vi "main 7th.vi"() -> ()   [LabVIEW 2015]
panel:
  out "3":u32
  out "1":u32
  out "2":u32
  out "5":u32
  out "4":u32
  out "element":u16[][](array[numeric])
  out "From OD fit?":bool
  in  "Current file num":i32
  in  "Fitting Results Save Path":string[](array[string])
  in  "Initial guess values":dbl[](array[numeric])
  out "Latest image data":dbl[][](array[numeric])
  in  "Fitting Type":u16(ring)
  in  "Force Guess?":bool
  in  "milliseconds to wait":u32
  out "best fit parameters":dbl[](array[numeric])
  in  "Reset process index":bool
  out "ROI Height":u32
  out "ROI Width":u32
  out "OD image":u16[][](graph)
  out "Process Index":i32
  out "External Trigger":bool
  out "XY图":cluster{i32[], dbl[]}[](graph)
  in  "OD fit":bool
  in  "OD num":i32
  out "Fit Done":bool
  in  "Exit":bool
  out "XY图 2":cluster{i32[], dbl[]}[](graph)
  in  "Fit":bool
  in  "Open File":bool
  in  "Auto Fit":bool
  in  "Stop":bool
  in  "Aquire":bool
  in  "Fitting Config":bool
  in  "Camera Config":bool
  in  "Initialize":bool
  in  "Live Image Display":refnum<k7>(container)
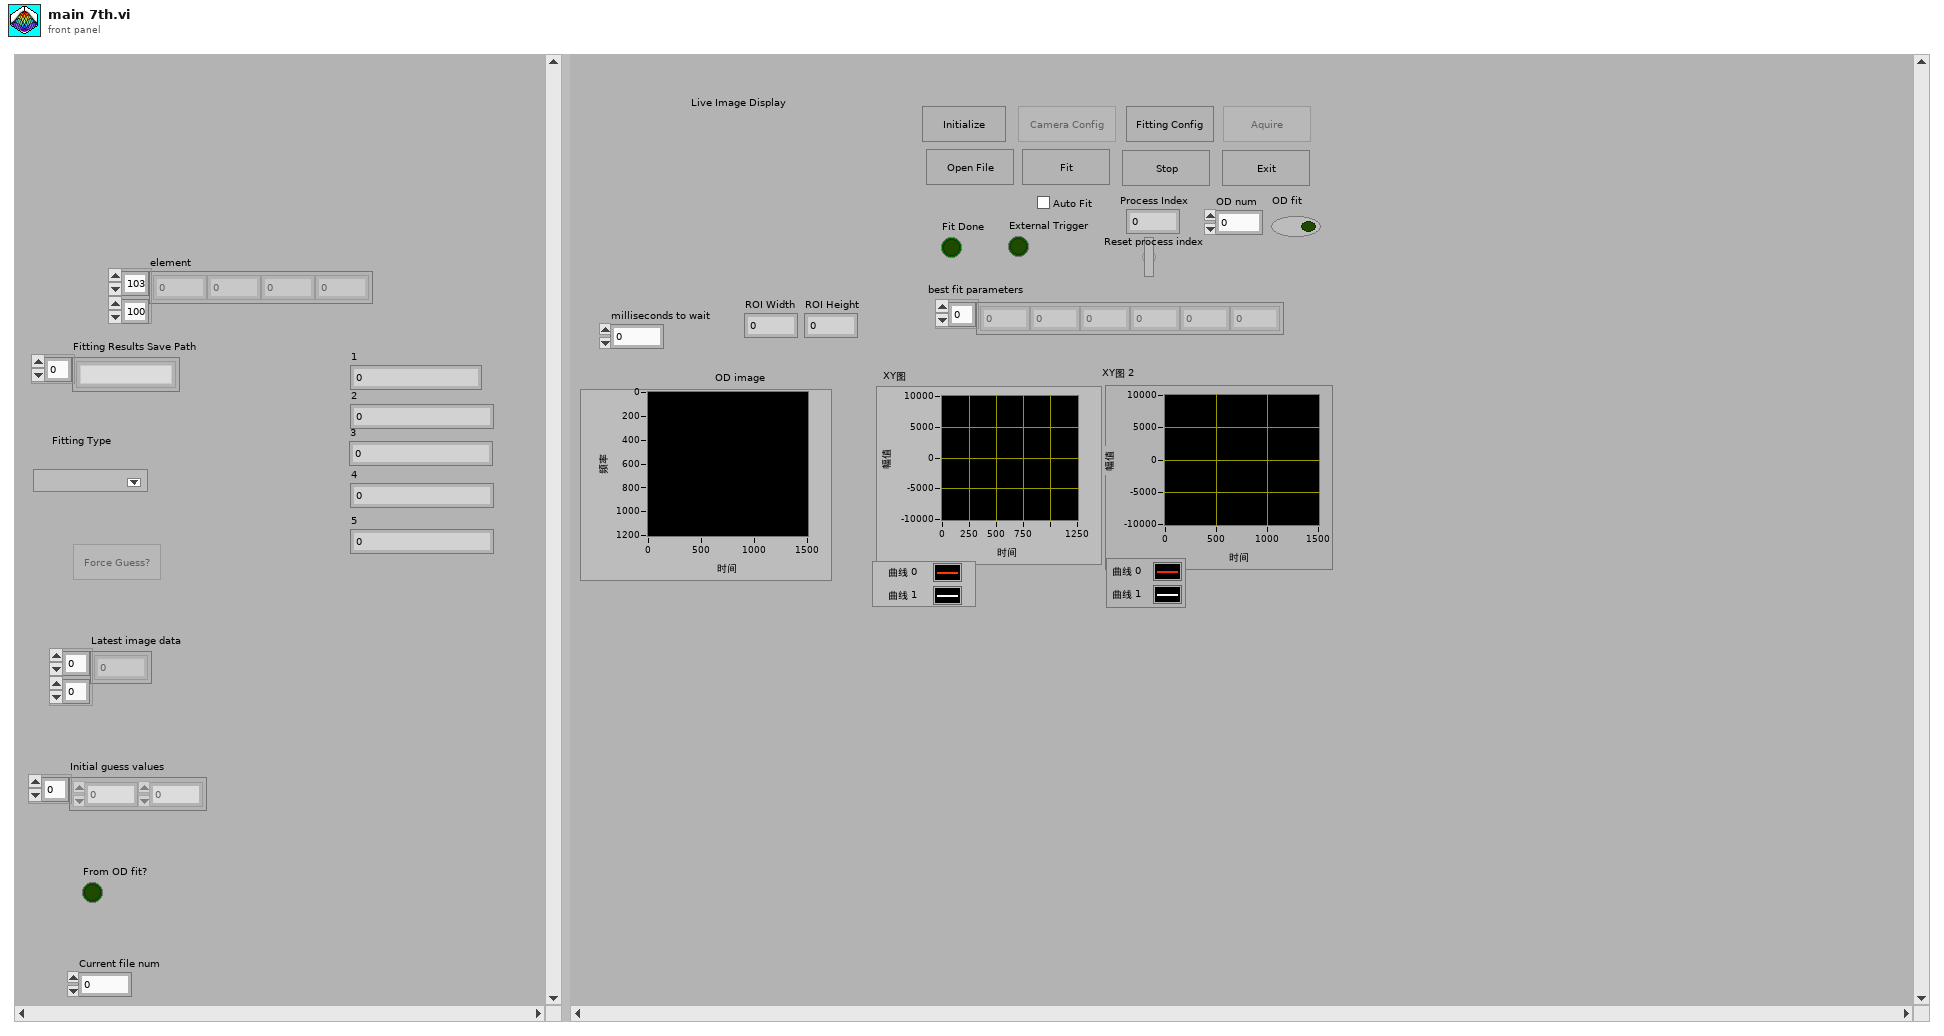
[diagram p1: front panel]
types:
  T1 = enum8{"Enabled", "Disabled", "Disabled and Grayed Out"}
  T2 = typedef "Image Type" = u32
  T3 = typedef "IMAQ Image.ctl" = refnum<image>
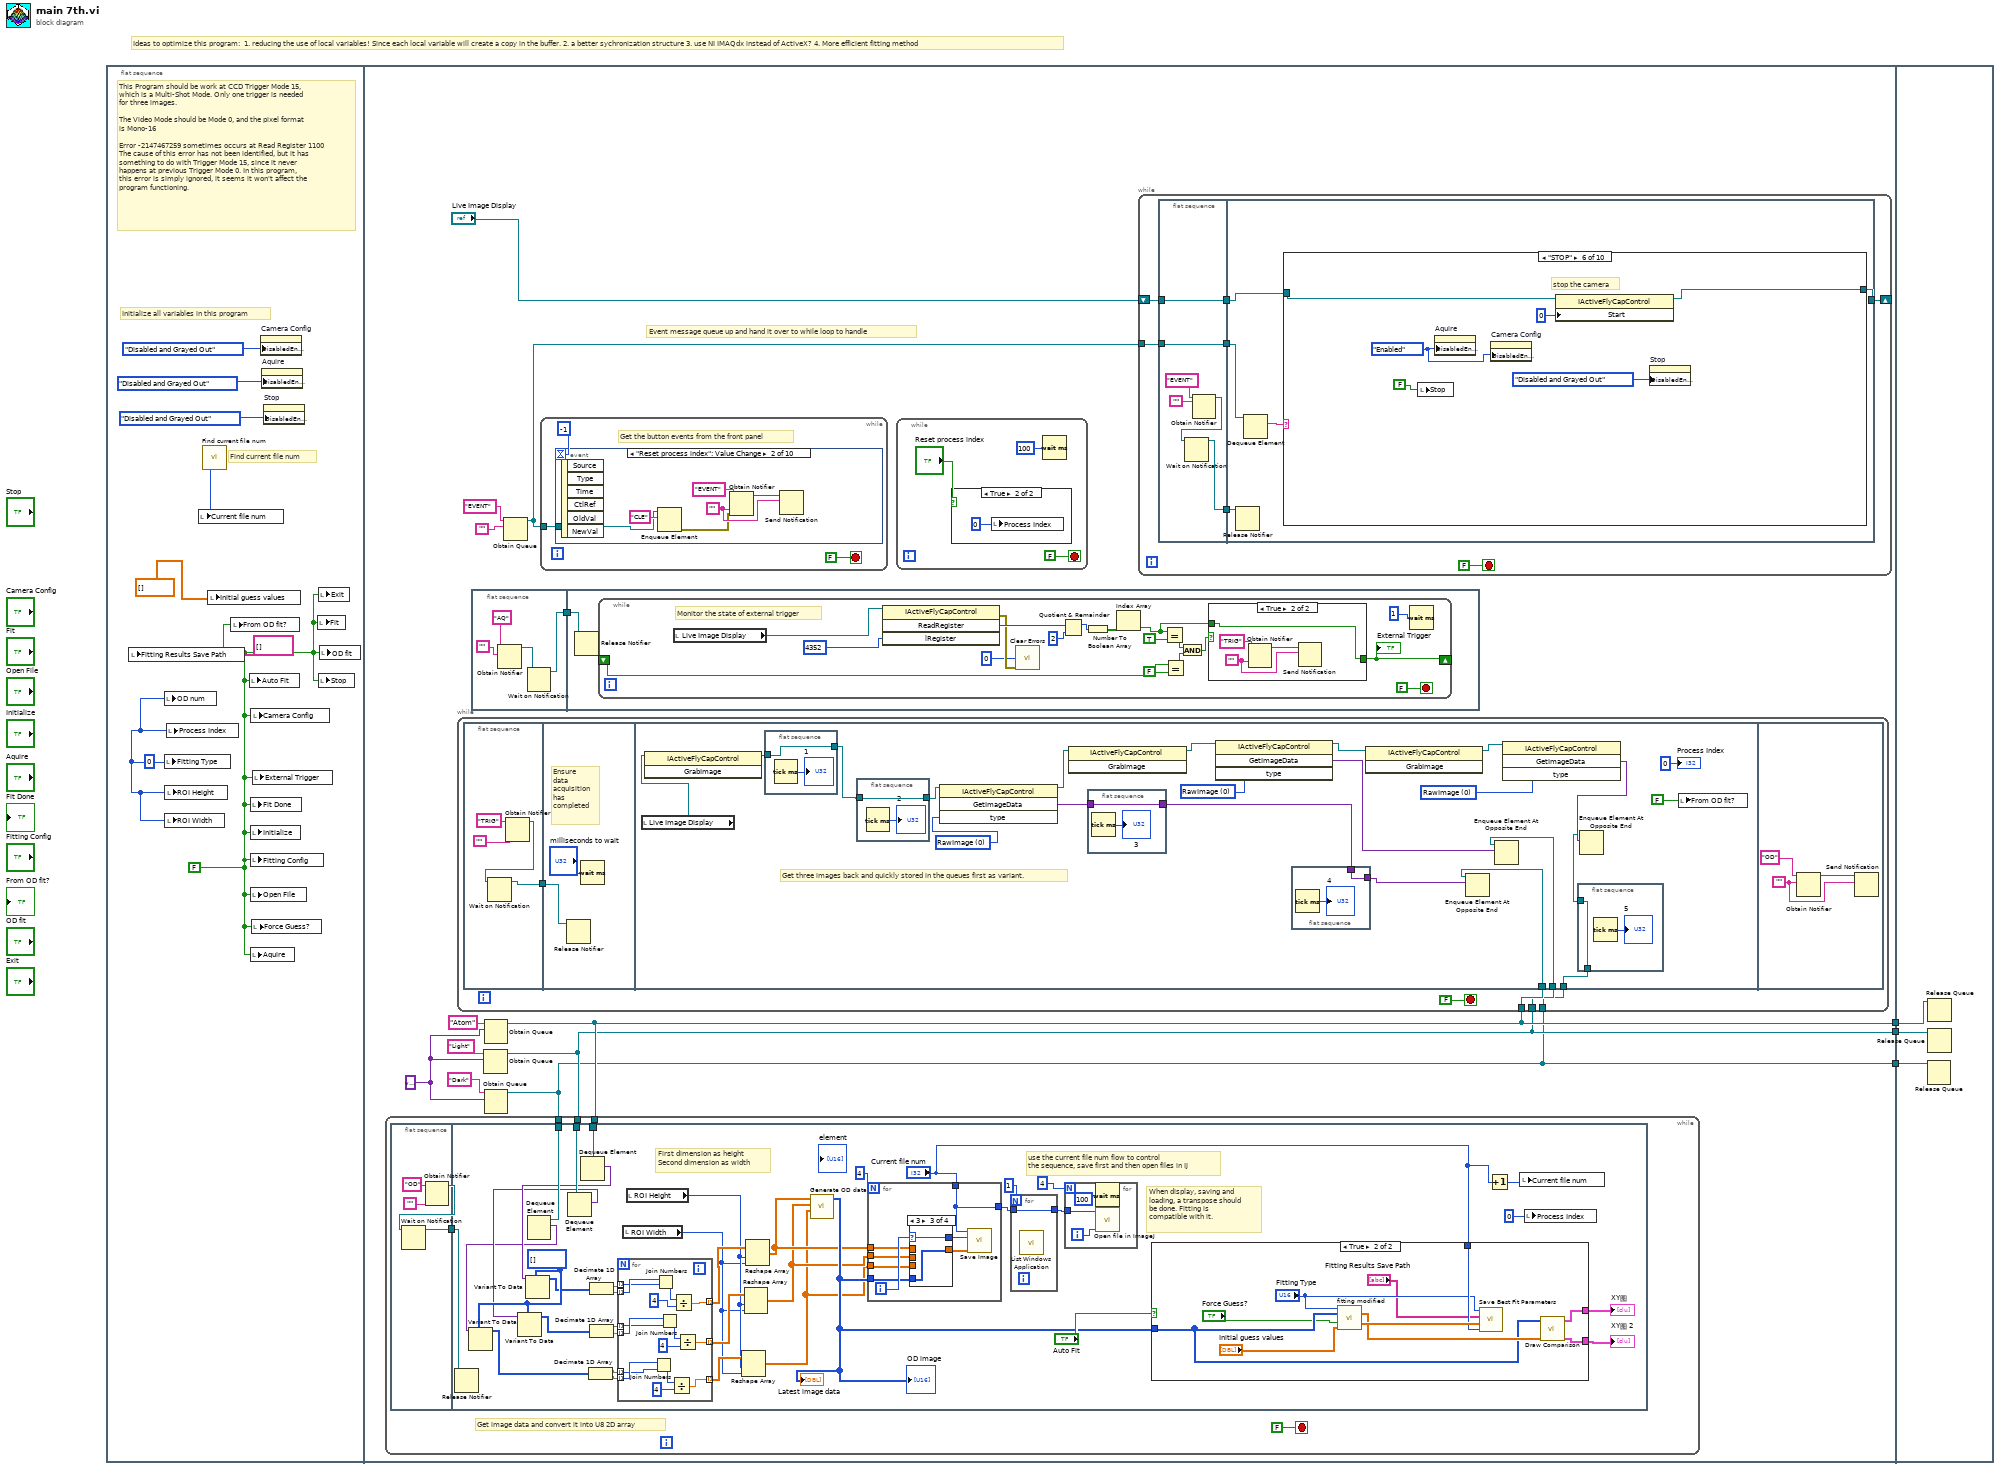
[diagram p0: block diagram]
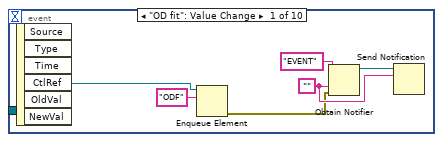
[diagram p2: hidden frame]
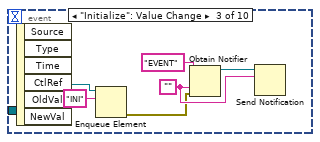
[diagram p3: hidden frame]
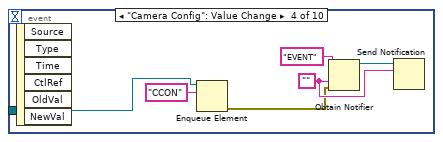
[diagram p4: hidden frame]
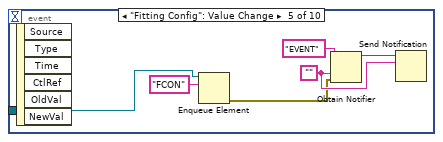
[diagram p5: hidden frame]
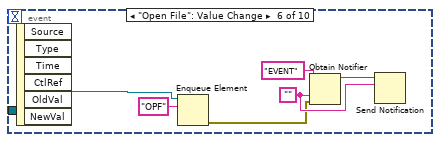
[diagram p6: hidden frame]
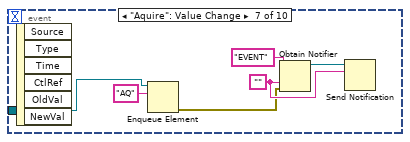
[diagram p7: hidden frame]
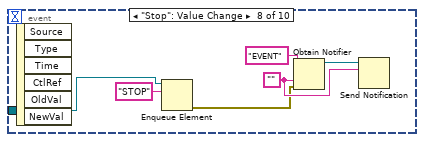
[diagram p8: hidden frame]
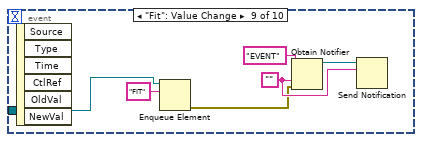
[diagram p9: hidden frame]
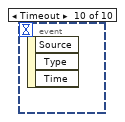
[diagram p10: hidden frame]
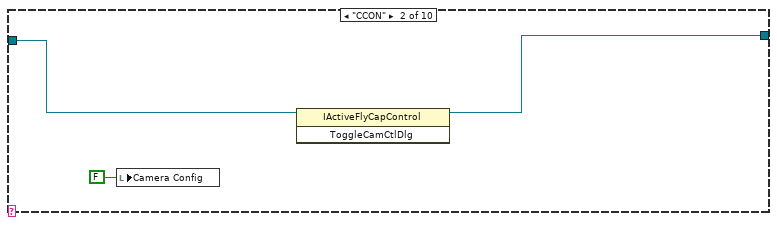
[diagram p12: hidden frame]
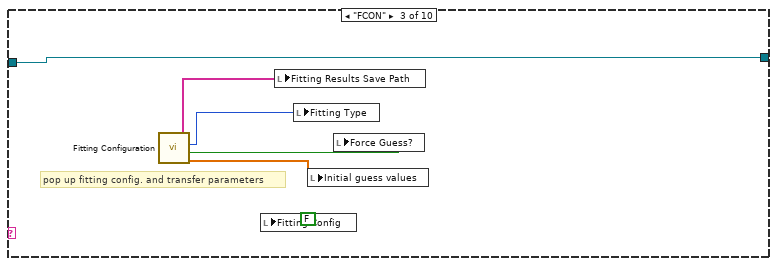
[diagram p13: hidden frame]
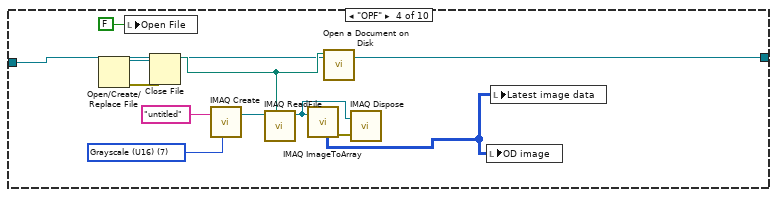
[diagram p14: hidden frame]
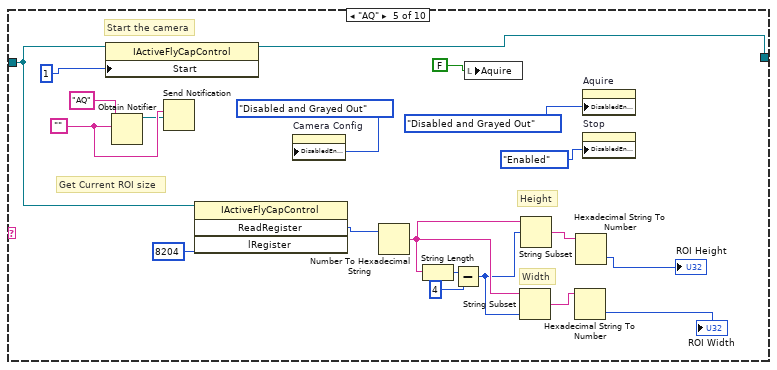
[diagram p15: hidden frame]
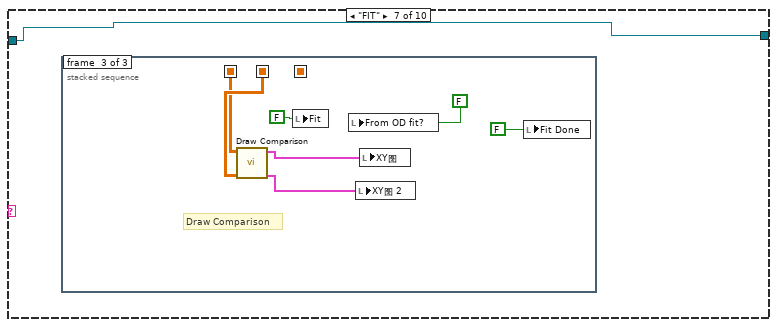
[diagram p16: hidden frame]
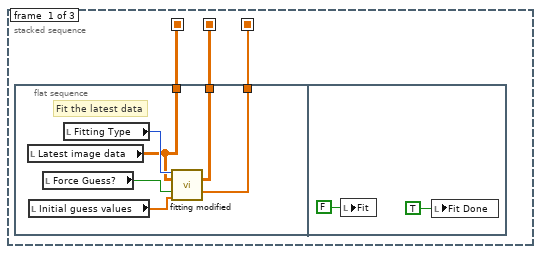
[diagram p17: hidden frame]
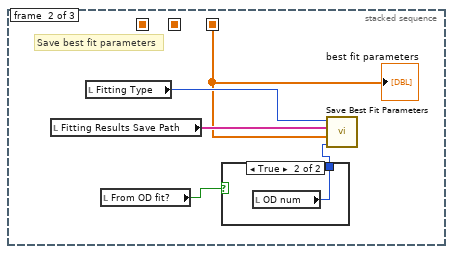
[diagram p18: hidden frame]
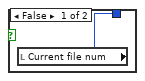
[diagram p19: hidden frame]
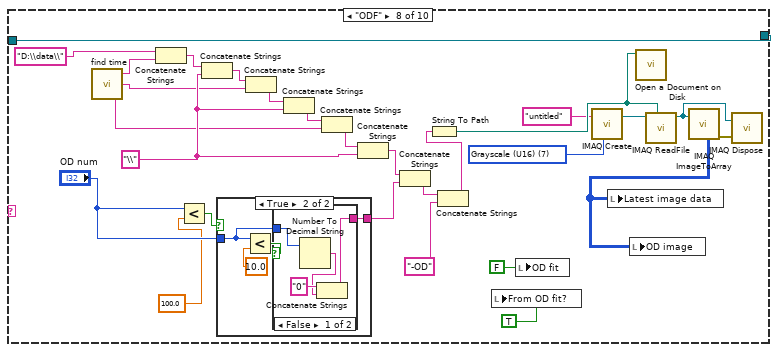
[diagram p20: hidden frame]
diagram:
  # "Ideas to optimize this program:  1. reducing the use of local variables! Since each local variable will create a copy in the buffer. 2. a better sychronization structure 3. use NI IMAQdx instead of ActiveX? 4. More efficient fitting method"
  n1 = flat-sequence {
    tunnel: [w19] -> w3
    tunnel: [w18] -> w2
    tunnel: [w17] -> w1
    tunnel: w3 -> [w405]
    tunnel: w2 -> [w404]
    tunnel: w1 -> [w403]
    frame #0 {
      w7 = 0 ("OD num")
      w5 = FALSE ("Aquire")
      # "This Program should be work at CCD Trigger Mode 15,\nwhich is a Multi-Shot Mode. Only one trigger is needed\nfor three images. \n\nThe Video Mode should be Mode 0, and the pixel format\nis Mono-16\n\nError -2147467259 sometimes occurs at Read Register 1100\nThe cause of this error has not been identified, but it has\nsomething to do with Trigger Mode 15, since it never \nhappens at previous Trigger Mode 0. In this program,\nthis error is simply ignored, it seems it won't affect the \nprogram functioning."
      # "Find current file num"
      # "Initialize all variables in this program"
      n2 = local write "Fitting Results Save Path"(string[] [] ("Fitting Results Save Path")) -> ()
      n3 = local write "OD num"(w7) -> ()
      n4 = local write "Fitting Type"(w7) -> ()
      n5 = local write "ROI Height"(w7) -> ()
      n6 = local write "ROI Width"(w7) -> ()
      n7 = local write "Process Index"(w7) -> ()
      n8 = call "Find current file num.vi"() -> ("Current File Num"=w4:u16)  [unwired: 2 in]
      n9 = local write "Current file num"(w4) -> ()
      n10 = local write "Initial guess values"(dbl[] [] ("Best fit parameters")) -> ()
      n11 = local write "From OD fit?"(w5) -> ()
      n12 = local write "Auto Fit"(w5) -> ()
      n13 = local write "Fit Done"(w5) -> ()
      n14 = local write "Initialize"(w5) -> ()
      n15 = local write "Fitting Config"(w5) -> ()
      n16 = local write "Open File"(w5) -> ()
      n17 = local write "Aquire"(w5) -> ()
      n18 = local write "Camera Config"(w5) -> ()
      n19 = local write "Force Guess?"(w5) -> ()
      n20 = local write "External Trigger"(w5) -> ()
      n21 = property on="Camera Config" class="Bool (strict)"("DisabledEnum"=T1."Disabled and Grayed Out" ("禁用")) -> ()  [unwired: 2 in, 2 out]
      n22 = property on="Aquire" class="Bool (strict)"("DisabledEnum"=T1."Disabled and Grayed Out" ("禁用")) -> ()  [unwired: 2 in, 2 out]
      n23 = property on="Stop" class="Bool (strict)"("DisabledEnum"=T1."Disabled and Grayed Out" ("禁用")) -> ()  [unwired: 2 in, 2 out]
      n24 = local write "Fit"(w5) -> ()
      n25 = local write "Exit"(w5) -> ()
      n26 = local write "Stop"(w5) -> ()
      n27 = local write "OD fit"(w5) -> ()
    }
    frame #1 {
      w13 = variant
      # "Event message queue up and hand it over to while loop to handle"
      n28 = flat-sequence {
        tunnel: [w329] -> w23
        tunnel: w23 -> [w333]
        frame #0 {
          n29 = Obtain Notifier(name (unnamed)="AQ" ("名称（未命名）"), notification data type="") -> (notifier out=w331:refnum<notifier>)  [unwired: 2 in, 2 out]
          n30 = Wait on Notification(notifier=w331) -> (notifier out=w329:refnum<notifier>)  [unwired: 3 in, 3 out]
        }
        frame #1 {
          n31 = Release Notifier(notifier=w333) -> ()  [unwired: 2 in, 3 out]
          n32 = while {
            shift-right: [w338] -> _
            shift-left: _ -> [w337]
            stop <- FALSE stop-if-true
            # "Monitor the state of external trigger"
            n33 = local read "Live Image Display"() -> (w351:refnum<k7>)
            n34 = invoke class="IActiveFlyCapControl" method="ReadRegister"(reference=w351, "lRegister"=u32 4352) -> (error out=w335:errorcluster, "ReadRegister"=w349:u32)  [unwired: 2 in, 2 out]
            n35 = call <vilib>:"Clear Errors.vi"("error in (no error)"=w335, "specific error code to clear (0: all)"=0) -> ()  [unwired: 4 in, 2 out]
            n36 = Quotient & Remainder(x=w349, y=u32 2) -> (x-y*floor(x/y)=w347:u32)  [unwired: 1 out]
            n37 = Number To Boolean Array(number=w347) -> (Boolean array=w346:bool[])
            n38 = Index Array(array=w346) -> (element=w340:bool)  [unwired: 1 in]
            n39 = Equal?(x=w340, y=TRUE) -> (x = y?=w342:bool)
            n40 = Equal?(x=w337, y=FALSE) -> (x = y?=w343:bool)
            n41 = And(x=w342, y=w343) -> (x .and. y?=w341:bool)
            n42 = case shown="True" w341 {
              tunnel: w340 -> [w352 w353]
              tunnel: [w352 w353] -> w338
              frame False {
              }
              frame True {
                w354 = ""
                n43 = Obtain Notifier(name (unnamed)="TRIG" ("名称（未命名）"), notification data type=w354) -> (notifier out=w355:refnum<notifier>)  [unwired: 2 in, 2 out]
                n44 = Send Notification(notification=w354, notifier=w355) -> ()  [unwired: 1 in, 2 out]
              }
            }
            "External Trigger" <- w338
            n45 = Wait (ms)(milliseconds to wait=u32 1) -> ()  [unwired: 1 out]
          }
        }
      }
      n46 = Obtain Queue(name (unnamed)="Light" ("名称（未命名）"), element data type=w13) -> (queue out=w18:refnum<queue>)  [unwired: 3 in, 2 out]
      n47 = Obtain Queue(name (unnamed)="Atom" ("名称（未命名）"), element data type=w13) -> (queue out=w19:refnum<queue>)  [unwired: 3 in, 2 out]
      n48 = Obtain Queue(name (unnamed)="Dark" ("名称（未命名）"), element data type=w13) -> (queue out=w17:refnum<queue>)  [unwired: 3 in, 2 out]
      n49 = while {
        tunnel: w19 -> [w238]
        tunnel: w18 -> [w237]
        tunnel: w17 -> [w236]
        stop <- FALSE stop-if-true
        # "Get image data and convert it into U8 2D array"
        n50 = flat-sequence {
          tunnel: [w240] -> w239
          tunnel: w239 -> [w249]
          tunnel: w238 -> [w279]
          tunnel: w237 -> [w278]
          tunnel: w236 -> [w277]
          frame #0 {
            n51 = Obtain Notifier(name (unnamed)="OD" ("名称（未命名）"), notification data type="") -> (notifier out=w241:refnum<notifier>)  [unwired: 2 in, 2 out]
            n52 = Wait on Notification(notifier=w241) -> (notifier out=w240:refnum<notifier>)  [unwired: 3 in, 3 out]
          }
          frame #1 {
            w252 = u8[] []
            # "When display, saving and \nloading, a transpose should\nbe done. Fitting is \ncompatible with it."
            # "First dimension as height\nSecond dimension as width"
            # "use the current file num flow to control \nthe sequence, save first and then open files in IJ"
            n53 = Release Notifier(notifier=w249) -> ()  [unwired: 2 in, 3 out]
            n54 = Dequeue Element(queue=w277) -> (element=w250:variant)  [unwired: 2 in, 3 out]
            n55 = Variant To Data(type=w252, Variant=w250) -> (data=w246:u8[])  [unwired: 1 in, 1 out]
            n56 = Dequeue Element(queue=w278) -> (element=w251:variant)  [unwired: 2 in, 3 out]
            n57 = Variant To Data(type=w252, Variant=w251) -> (data=w247:u8[])  [unwired: 1 in, 1 out]
            n58 = Dequeue Element(queue=w279) -> (element=w253:variant)  [unwired: 2 in, 3 out]
            n59 = Variant To Data(type=w252, Variant=w253) -> (data=w248:u8[])  [unwired: 1 in, 1 out]
            n60 = Decimate 1D Array(w246) -> (w261:u8[], w260:u8[])
            n61 = Decimate 1D Array(w248) -> (w265:u8[], w264:u8[])
            n62 = Decimate 1D Array(w247) -> (w263:u8[], w262:u8[])
            n63 = for {
              tunnel: [w293] -> w259 mode=indexing
              tunnel: w265 -> [w283] mode=indexing
              tunnel: w264 -> [w284] mode=indexing
              tunnel: w263 -> [w285] mode=indexing
              tunnel: w262 -> [w286] mode=indexing
              tunnel: w261 -> [w287] mode=indexing
              tunnel: w260 -> [w288] mode=indexing
              tunnel: [w282] -> w258 mode=indexing
              tunnel: [w281] -> w257 mode=indexing
              n64 = Join Numbers(hi=w288, lo=w287) -> ((hi.lo)=w290:u16)
              n65 = Join Numbers(hi=w284, lo=w283) -> ((hi.lo)=w295:u16)
              n66 = Join Numbers(hi=w286, lo=w285) -> ((hi.lo)=w292:u16)
              n67 = Divide(x=w290, y=u16 4) -> (x/y=w281:dbl)
              n68 = Divide(x=w295, y=u16 4) -> (x/y=w293:dbl)
              n69 = Divide(x=w292, y=u16 4) -> (x/y=w282:dbl)
            }
            n70 = local read "ROI Width"() -> (w244:u32)
            n71 = local read "ROI Height"() -> (w245:u32)
            n72 = Reshape Array(w257, w245, w244) -> (w254:dbl[][])
            n73 = Reshape Array(w258, w245, w244) -> (w255:dbl[][])
            n74 = Reshape Array(w259, w245, w244) -> (w256:dbl[][])
            n75 = call "Generate OD data.vi"("dark"=w254, "light"=w255, "atom"=w256) -> ("OD image"=w273:u16[][])  [unwired: 3 in]
            "OD image" <- w273
            "Latest image data" <- w273
            n76 = for {
              N: 4 -> [_]
              tunnel: w256 -> [w319]
              tunnel: w255 -> [w318]
              tunnel: w254 -> [w317]
              tunnel: w273 -> [w316]
              tunnel: "Current file num" -> [w313]
              tunnel: [w313] -> w266
              i -> [w320]
              n77 = case shown="3" w320 {
                selector: w320 -> [w322 w324 w326 w328]
                tunnel: w319 -> [w321 _ _ _]
                tunnel: w318 -> [_ _ _ w327]
                tunnel: w317 -> [_ w323 _ _]
                tunnel: w316 -> [_ _ w325 _]
                tunnel: [w322 w324 w326 w328] -> w315
                tunnel: [w321 w323 w325 w327] -> w314
                frame 0, Default {
                }
                frame 2 {
                }
                frame 3 {
                }
                frame 1 {
                }
              }
              n78 = call "Save Image.vi"("Data"=w314, "Process Index"=w315, "Current File Num"=w313) -> ()  [unwired: 9 in]
            }
            n79 = for {
              N: 1 -> [_]
              tunnel: w266 -> [w296]
              tunnel: [w296] -> w268
              n80 = call "List Windows Application.vi"() -> ()  [unwired: 1 in]
            }
            n81 = for {
              N: 4 -> [_]
              tunnel: w268 -> [w299]
              i -> [w298]
              n82 = Wait (ms)(milliseconds to wait=u32 100) -> ()  [unwired: 1 out]
              n83 = call "Open file in ImageJ.vi"("Process Index"=w298, "Current File Num"=w299) -> ()  [unwired: 10 in]
            }
            n84 = case shown="True" "Auto Fit" {
              tunnel: w273 -> [w302 w309]
              tunnel: "Current file num" -> [_ w311]
              tunnel: [w301 w308] -> w274
              tunnel: [w300 w307] -> w275
              frame False {
                n85 = call "Draw Comparison.vi"("Best Fit"=w302, "Raw Data"=w302) -> ("Vertical Comparison"=w300:cluster{i32[], dbl[]}[], "Horizontal Comparison"=w301:cluster{i32[], dbl[]}[])  [unwired: 7 in]
              }
              frame True {
                n86 = call "fitting modified.vi"("fitting type"="Fitting Type", "2D data"=w309, "force guess?"="Force Guess?", "intial guess value"="Initial guess values") -> ("best fit"=w310:dbl[][], "best fit parameters"=w312:dbl[])  [unwired: 8 in, 2 out]
                n87 = call "Save Best Fit Parameters.vi"("Current File Num"=w311, "Best Fit Parameters"=w312, "Fitting Results Save Path"="Fitting Results Save Path", "Fitting Type"="Fitting Type") -> ()  [unwired: 8 in]
                n88 = call "Draw Comparison.vi"("Best Fit"=w310, "Raw Data"=w309) -> ("Vertical Comparison"=w307:cluster{i32[], dbl[]}[], "Horizontal Comparison"=w308:cluster{i32[], dbl[]}[])  [unwired: 7 in]
              }
            }
            "XY图" <- w274
            "XY图 2" <- w275
            n89 = Increment(x="Current file num") -> (x+1=w272:i32)
            n90 = local write "Current file num"(w272) -> ()
            n91 = local write "Process Index"(0 ("Process Index")) -> ()
          }
        }
      }
      n92 = while {
        tunnel: w19 -> [w360]
        tunnel: w18 -> [w359]
        tunnel: w17 -> [w358]
        stop <- FALSE stop-if-true
        n93 = flat-sequence {
          tunnel: [w362] -> w361
          tunnel: w361 -> [w367]
          tunnel: w360 -> [w386]
          tunnel: w359 -> [w375]
          tunnel: w358 -> [w371]
          frame #0 {
            n94 = Obtain Notifier(name (unnamed)="TRIG" ("名称（未命名）"), notification data type="") -> (notifier out=w363:refnum<notifier>)  [unwired: 2 in, 2 out]
            n95 = Wait on Notification(notifier=w363) -> (notifier out=w362:refnum<notifier>)  [unwired: 3 in, 3 out]
          }
          frame #1 {
            # "Ensure\ndata\nacquisition\nhas \ncompleted"
            n96 = Release Notifier(notifier=w367) -> ()  [unwired: 2 in, 3 out]
            n97 = Wait (ms)(milliseconds to wait="milliseconds to wait") -> ()  [unwired: 1 out]
          }
          frame #2 {
            w368 = 0 items=["RawImage", "ColorProcessedImage"] ("type")
            w369 = 0 items=["RawImage", "ColorProcessedImage"] ("type")
            w389 = 0 items=["RawImage", "ColorProcessedImage"] ("type")
            # "Get three images back and quickly stored in the queues first as variant."
            n98 = local read "Live Image Display"() -> (w387:refnum<k7>)
            n99 = invoke class="IActiveFlyCapControl" method="GrabImage"(reference=w387) -> (reference out=w383:refnum<k7>)  [unwired: 2 in, 2 out]
            n100 = flat-sequence {
              tunnel: [w392] -> w380
              tunnel: w383 -> [w392]
              frame #0 {
                n101 = Tick Count (ms)() -> (millisecond timer value=→"1":u32)
              }
            }
            n102 = flat-sequence {
              tunnel: w380 -> [w394]
              tunnel: [w394] -> w384
              frame #0 {
                n103 = Tick Count (ms)() -> (millisecond timer value=→"2":u32)
              }
            }
            n104 = invoke class="IActiveFlyCapControl" method="GetImageData"(reference=w384, "type"=w389) -> (reference out=w379:refnum<k7>, "GetImageData"=w382:variant)  [unwired: 2 in, 2 out]
            n105 = invoke class="IActiveFlyCapControl" method="GrabImage"(reference=w379) -> (reference out=w378:refnum<k7>)  [unwired: 2 in, 2 out]
            n106 = flat-sequence {
              tunnel: [w390] -> w381
              tunnel: w382 -> [w390]
              frame #0 {
                n107 = Tick Count (ms)() -> (millisecond timer value=→"3":u32)
              }
            }
            n108 = invoke class="IActiveFlyCapControl" method="GetImageData"(reference=w378, "type"=w369) -> (reference out=w377:refnum<k7>, "GetImageData"=w376:variant)  [unwired: 2 in, 2 out]
            n109 = flat-sequence {
              tunnel: w381 -> [w399]
              tunnel: [w399] -> w385
              frame #0 {
                n110 = Tick Count (ms)() -> (millisecond timer value=→"4":u32)
              }
            }
            n111 = invoke class="IActiveFlyCapControl" method="GrabImage"(reference=w377) -> (reference out=w374:refnum<k7>)  [unwired: 2 in, 2 out]
            n112 = Enqueue Element At Opposite End(queue=w386, element=w385) -> ()  [unwired: 2 in, 3 out]
            n113 = Enqueue Element At Opposite End(queue=w375, element=w376) -> ()  [unwired: 2 in, 3 out]
            n114 = invoke class="IActiveFlyCapControl" method="GetImageData"(reference=w374, "type"=w368) -> ("GetImageData"=w373:variant)  [unwired: 2 in, 3 out]
            n115 = flat-sequence {
              tunnel: w371 -> [w396]
              tunnel: [w396] -> w370
              frame #0 {
                n116 = Tick Count (ms)() -> (millisecond timer value=→"5":u32)
              }
            }
            n117 = Enqueue Element At Opposite End(queue=w370, element=w373) -> ()  [unwired: 2 in, 3 out]
            n118 = local write "From OD fit?"(FALSE ("From OD fit?")) -> ()
            "Process Index" <- 0 ("Process Index")
          }
          frame #3 {
            w400 = ""
            n119 = Obtain Notifier(name (unnamed)="OD" ("名称（未命名）"), notification data type=w400) -> (notifier out=w402:refnum<notifier>)  [unwired: 2 in, 2 out]
            n120 = Send Notification(notification=w400, notifier=w402) -> ()  [unwired: 1 in, 2 out]
          }
        }
      }
      n121 = Obtain Queue(name (unnamed)="EVENT" ("名称（未命名）"), element data type="") -> (queue out=w14:refnum<queue>)  [unwired: 3 in, 2 out]
      n122 = while {
        tunnel: w14 -> [w24]
        stop <- FALSE stop-if-true
        # "Get the button events from the front panel"
        n123 = event shown="[1] \"Reset process index\": Value Change" {
          selector: _ -> [_ _ _ _ _ _ _ _ _ _]
          dyn-events: _ -> [_ _ _ _ _ _ _ _ _ _]
          timeout: -1 -> [_ _ _ _ _ _ _ _ _ _]
          tunnel: w24 -> [w27 w33 w40 w45 w51 w57 w63 w69 w75 _]
          event "OD fit": Value Change {
            w30 = ""
            n124 = event-data() -> ()  [unwired: 1 in, 6 out]
            n125 = Enqueue Element(queue=w27, element="ODF") -> (error out=w28:errorcluster)  [unwired: 2 in, 2 out]
            n126 = Obtain Notifier(name (unnamed)="EVENT" ("名称（未命名）"), notification data type=w30, error in (no error)=w28) -> (notifier out=w31:refnum<notifier>)  [unwired: 1 in, 2 out]
            n127 = Send Notification(notification=w30, notifier=w31) -> ()  [unwired: 1 in, 2 out]
          }
          event "Reset process index": Value Change {
            w36 = ""
            n128 = event-data() -> ()  [unwired: 1 in, 6 out]
            n129 = Enqueue Element(queue=w33, element="CLE") -> (error out=w34:errorcluster)  [unwired: 2 in, 2 out]
            n130 = Obtain Notifier(name (unnamed)="EVENT" ("名称（未命名）"), notification data type=w36, error in (no error)=w34) -> (notifier out=w37:refnum<notifier>)  [unwired: 1 in, 2 out]
            n131 = Send Notification(notification=w36, notifier=w37) -> ()  [unwired: 1 in, 2 out]
          }
          event "Initialize": Value Change {
            w42 = ""
            n132 = event-data() -> ()  [unwired: 1 in, 6 out]
            n133 = Enqueue Element(queue=w40, element="INI") -> (error out=w39:errorcluster)  [unwired: 2 in, 2 out]
            n134 = Obtain Notifier(name (unnamed)="EVENT" ("名称（未命名）"), notification data type=w42, error in (no error)=w39) -> (notifier out=w43:refnum<notifier>)  [unwired: 1 in, 2 out]
            n135 = Send Notification(notification=w42, notifier=w43) -> ()  [unwired: 1 in, 2 out]
          }
          event "Camera Config": Value Change {
            w48 = ""
            n136 = event-data() -> ()  [unwired: 1 in, 6 out]
            n137 = Enqueue Element(queue=w45, element="CCON") -> (error out=w46:errorcluster)  [unwired: 2 in, 2 out]
            n138 = Obtain Notifier(name (unnamed)="EVENT" ("名称（未命名）"), notification data type=w48, error in (no error)=w46) -> (notifier out=w49:refnum<notifier>)  [unwired: 1 in, 2 out]
            n139 = Send Notification(notification=w48, notifier=w49) -> ()  [unwired: 1 in, 2 out]
          }
          event "Fitting Config": Value Change {
            w54 = ""
            n140 = event-data() -> ()  [unwired: 1 in, 6 out]
            n141 = Enqueue Element(queue=w51, element="FCON") -> (error out=w52:errorcluster)  [unwired: 2 in, 2 out]
            n142 = Obtain Notifier(name (unnamed)="EVENT" ("名称（未命名）"), notification data type=w54, error in (no error)=w52) -> (notifier out=w55:refnum<notifier>)  [unwired: 1 in, 2 out]
            n143 = Send Notification(notification=w54, notifier=w55) -> ()  [unwired: 1 in, 2 out]
          }
          event "Open File": Value Change {
            w60 = ""
            n144 = event-data() -> ()  [unwired: 1 in, 6 out]
            n145 = Enqueue Element(queue=w57, element="OPF") -> (error out=w58:errorcluster)  [unwired: 2 in, 2 out]
            n146 = Obtain Notifier(name (unnamed)="EVENT" ("名称（未命名）"), notification data type=w60, error in (no error)=w58) -> (notifier out=w61:refnum<notifier>)  [unwired: 1 in, 2 out]
            n147 = Send Notification(notification=w60, notifier=w61) -> ()  [unwired: 1 in, 2 out]
          }
          event "Aquire": Value Change {
            w66 = ""
            n148 = event-data() -> ()  [unwired: 1 in, 6 out]
            n149 = Enqueue Element(queue=w63, element="AQ") -> (error out=w64:errorcluster)  [unwired: 2 in, 2 out]
            n150 = Obtain Notifier(name (unnamed)="EVENT" ("名称（未命名）"), notification data type=w66, error in (no error)=w64) -> (notifier out=w67:refnum<notifier>)  [unwired: 1 in, 2 out]
            n151 = Send Notification(notification=w66, notifier=w67) -> ()  [unwired: 1 in, 2 out]
          }
          event "Stop": Value Change {
            w72 = ""
            n152 = event-data() -> ()  [unwired: 1 in, 6 out]
            n153 = Enqueue Element(queue=w69, element="STOP") -> (error out=w70:errorcluster)  [unwired: 2 in, 2 out]
            n154 = Obtain Notifier(name (unnamed)="EVENT" ("名称（未命名）"), notification data type=w72, error in (no error)=w70) -> (notifier out=w73:refnum<notifier>)  [unwired: 1 in, 2 out]
            n155 = Send Notification(notification=w72, notifier=w73) -> ()  [unwired: 1 in, 2 out]
          }
          event "Fit": Value Change {
            w78 = ""
            n156 = event-data() -> ()  [unwired: 1 in, 6 out]
            n157 = Enqueue Element(queue=w75, element="FIT") -> (error out=w76:errorcluster)  [unwired: 2 in, 2 out]
            n158 = Obtain Notifier(name (unnamed)="EVENT" ("名称（未命名）"), notification data type=w78, error in (no error)=w76) -> (notifier out=w79:refnum<notifier>)  [unwired: 1 in, 2 out]
            n159 = Send Notification(notification=w78, notifier=w79) -> ()  [unwired: 1 in, 2 out]
          }
          event Timeout {
            n160 = event-data() -> ()  [unwired: 1 in, 3 out]
          }
        }
      }
      n161 = while {
        stop <- FALSE stop-if-true
        n162 = case shown="True" "Reset process index" {
          frame False {
          }
          frame True {
            n163 = local write "Process Index"(0 ("Process Index")) -> ()
          }
        }
        n164 = Wait (ms)(milliseconds to wait=u32 100 ("等待时间（毫秒）")) -> ()  [unwired: 1 out]
      }
      n165 = while {
        tunnel: w14 -> [w85]
        shift-right: [w81] -> _
        shift-left: "Live Image Display" -> [w82]
        stop <- FALSE stop-if-true
        n166 = flat-sequence {
          tunnel: [w90] -> w87
          tunnel: w85 -> [w89]
          tunnel: [w89] -> w84
          tunnel: [w88] -> w83
          tunnel: w82 -> [w88]
          tunnel: w87 -> [w98]
          tunnel: w84 -> [w97]
          tunnel: w83 -> [w95]
          tunnel: [w94] -> w81
          frame #0 {
            n167 = Obtain Notifier(name (unnamed)="EVENT" ("名称（未命名）"), notification data type="") -> (notifier out=w91:refnum<notifier>)  [unwired: 2 in, 2 out]
            n168 = Wait on Notification(notifier=w91) -> (notifier out=w90:refnum<notifier>)  [unwired: 3 in, 3 out]
          }
          frame #1 {
            n169 = Release Notifier(notifier=w98) -> ()  [unwired: 2 in, 3 out]
            n170 = Dequeue Element(queue=w97) -> (element=w96:string)  [unwired: 2 in, 3 out]
            n171 = case shown="\"STOP\"" w96 {
              tunnel: w95 -> [w99 w101 w103 w109 w120 w141 w146 w172 w214 w228]
              tunnel: [w99 w100 w103 w109 w131 w140 w146 w172 w215 w226] -> w94
              frame Default {
              }
              frame "CCON" {
                n172 = local write "Camera Config"(FALSE ("Camera Config")) -> ()
                n173 = invoke class="IActiveFlyCapControl" method="ToggleCamCtlDlg"(reference=w101) -> (reference out=w100:refnum<k7>)  [unwired: 2 in, 2 out]
              }
              frame "FCON" {
                # "pop up fitting config. and transfer parameters"
                n174 = call "Fitting Configuration.vi"() -> ("intial guess"=w108:dbl[], "Force Guess？"=w107:bool, "Fitting Type"=w105:u16, "Fitting Results Save Path"=w106:string[])  [unwired: 5 in]
                n175 = local write "Fitting Config"(FALSE ("Fitting Config")) -> ()
                n176 = local write "Fitting Results Save Path"(w106) -> ()
                n177 = local write "Fitting Type"(w105) -> ()
                n178 = local write "Initial guess values"(w108) -> ()
                n179 = local write "Force Guess?"(w107) -> ()
              }
              frame "OPF" {
                w111 = T2 7 items=["Grayscale (U8)", "Grayscale (I16)", "Grayscale (SGL)", "Complex (CSG)", "RGB (U32)", "HSL (U32)", "RGB (U64)", "Grayscale (U16)"] ("Image Type")
                n180 = Open/Create/Replace File() -> (refnum out=w118:refnum<file>, error out=w117:errorcluster)  [unwired: 6 in, 1 out]
                n181 = local write "Open File"(FALSE ("Open File")) -> ()
                n182 = Close File(refnum=w118, error in=w117) -> (path=w119:path)  [unwired: 1 out]
                n183 = call "IMAQ Create"("Image Name"="untitled", "Image Type"=w111) -> ("New Image"=w112:T3)  [unwired: 3 in, 1 out]
                n184 = call "IMAQ ReadFile"("File Path"=w119, "Image"=w112) -> ("Image Out"=w113:T3)  [unwired: 5 in, 4 out]
                n185 = call "IMAQ ImageToArray"("Image"=w113) -> ("Image Pixels (U16)"=w116:u16[][], "error out"=w114:errorcluster)  [unwired: 3 in, 3 out]
                n186 = call <vilib>:"Open a Document on Disk.vi"("document path"=w119) -> ()  [unwired: 6 in, 1 out]
                n187 = call "IMAQ Dispose"("Image"=w113, "error in (no error)"=w114) -> ()  [unwired: 4 in, 1 out]
                n188 = local write "OD image"(w116) -> ()
                n189 = local write "Latest image data"(w116) -> ()
              }
              frame "AQ" {
                w138 = ""
                # "Width"
                # "Height"
                # "Get Current ROI size"
                # "Start the camera"
                n190 = property class="IActiveFlyCapControl"(reference=w120, "Start"=1) -> (reference out=w131:refnum<k7>)  [unwired: 1 in, 1 out]
                n191 = Obtain Notifier(name (unnamed)="AQ" ("名称（未命名）"), notification data type=w138) -> (notifier out=w137:refnum<notifier>)  [unwired: 2 in, 2 out]
                n192 = Send Notification(notification=w138, notifier=w137) -> ()  [unwired: 1 in, 2 out]
                n193 = invoke class="IActiveFlyCapControl" method="ReadRegister"(reference=w120, "lRegister"=u32 8204) -> ("ReadRegister"=w122:u32)  [unwired: 2 in, 3 out]
                n194 = property on="Camera Config" class="Bool (strict)"("DisabledEnum"=T1."Disabled and Grayed Out" ("禁用")) -> ()  [unwired: 2 in, 2 out]
                n195 = Number To Hexadecimal String(2:w122) -> (0:w126:string)  [unwired: 1 in]
                n196 = String Length(string=w126) -> (length=w123:i32)
                n197 = Subtract(x=w123, y=4) -> (x-y=w125:i32)
                n198 = local write "Aquire"(FALSE ("Initialize")) -> ()
                n199 = String Subset(string=w126, length (rest)=w125) -> (substring=w128:string)  [unwired: 1 in]
                n200 = String Subset(string=w126, offset (0)=w125) -> (substring=w127:string)  [unwired: 1 in]
                n201 = Hexadecimal String To Number(string=w128) -> (number=→"ROI Width":u32)  [unwired: 2 in, 1 out]
                n202 = Hexadecimal String To Number(string=w127) -> (number=→"ROI Height":u32)  [unwired: 2 in, 1 out]
                n203 = property on="Aquire" class="Bool (strict)"("DisabledEnum"=T1."Disabled and Grayed Out" ("禁用")) -> ()  [unwired: 2 in, 2 out]
                n204 = property on="Stop" class="Bool (strict)"("DisabledEnum"=T1."Enabled" ("禁用")) -> ()  [unwired: 2 in, 2 out]
              }
              frame "STOP" {
                w145 = T1."Enabled" ("禁用")
                # "stop the camera"
                n205 = local write "Stop"(FALSE ("Initialize")) -> ()
                n206 = property on="Aquire" class="Bool (strict)"("DisabledEnum"=w145) -> ()  [unwired: 2 in, 2 out]
                n207 = property on="Camera Config" class="Bool (strict)"("DisabledEnum"=w145) -> ()  [unwired: 2 in, 2 out]
                n208 = property class="IActiveFlyCapControl"(reference=w141, "Start"=0) -> (reference out=w140:refnum<k7>)  [unwired: 1 in, 1 out]
                n209 = property on="Stop" class="Bool (strict)"("DisabledEnum"=T1."Disabled and Grayed Out" ("禁用")) -> ()  [unwired: 2 in, 2 out]
              }
              frame "FIT" {
                n210 = stacked-sequence {
                  seq-local: [w148 _ _] -> [_ _ w168]
                  seq-local: [w149 _ _] -> [_ _ w166]
                  seq-local: [w147 _ _] -> [_ w158 _]
                  frame #0 {
                    n211 = flat-sequence {
                      tunnel: [w152] -> w149
                      tunnel: [w151] -> w148
                      tunnel: [w150] -> w147
                      frame #0 {
                        # "Fit the latest data"
                        n212 = local read "Latest image data"() -> (w152:dbl[][])
                        n213 = local read "Initial guess values"() -> (w154:dbl[])
                        n214 = local read "Force Guess?"() -> (w155:bool)
                        n215 = local read "Fitting Type"() -> (w153:u16)
                        n216 = call "fitting modified.vi"("fitting type"=w153, "2D data"=w152, "force guess?"=w155, "intial guess value"=w154) -> ("best fit"=w151:dbl[][], "best fit parameters"=w150:dbl[])  [unwired: 8 in, 2 out]
                      }
                      frame #1 {
                        n217 = local write "Fit"(FALSE ("Fit")) -> ()
                        n218 = local write "Fit Done"(TRUE ("Fit Done")) -> ()
                      }
                    }
                  }
                  frame #1 {
                    # "Save best fit parameters"
                    n219 = local read "Fitting Results Save Path"() -> (w161:string[])
                    n220 = local read "Fitting Type"() -> (w162:u16)
                    n221 = local read "From OD fit?"() -> (w160:bool)
                    n222 = case shown="True" w160 {
                      tunnel: [w163 w164] -> w159
                      frame False {
                        n223 = local read "Current file num"() -> (w163:i32)
                      }
                      frame True {
                        n224 = local read "OD num"() -> (w164:i32)
                      }
                    }
                    n225 = call "Save Best Fit Parameters.vi"("Current File Num"=w159, "Best Fit Parameters"=w158, "Fitting Results Save Path"=w161, "Fitting Type"=w162) -> ()  [unwired: 8 in]
                    "best fit parameters" <- w158
                  }
                  frame #2 {
                    # "Draw Comparison"
                    n226 = call "Draw Comparison.vi"("Best Fit"=w168, "Raw Data"=w166) -> ("Vertical Comparison"=w170:cluster{i32[], dbl[]}[], "Horizontal Comparison"=w171:cluster{i32[], dbl[]}[])  [unwired: 7 in]
                    n227 = local write "Fit"(FALSE ("Initialize")) -> ()
                    n228 = local write "From OD fit?"(FALSE ("From OD fit?")) -> ()
                    n229 = local write "XY图 2"(w170) -> ()
                    n230 = local write "XY图"(w171) -> ()
                    n231 = local write "Fit Done"(FALSE ("Fit Done")) -> ()
                  }
                }
              }
              frame "ODF" {
                w193 = T2 7 items=["Grayscale (U8)", "Grayscale (I16)", "Grayscale (SGL)", "Complex (CSG)", "RGB (U32)", "HSL (U32)", "RGB (U64)", "Grayscale (U16)"] ("Image Type")
                w184 = "\\" ("字符串")
                n232 = call "find time.vi"() -> ("day"=w182:string, "month"=w179:string, "year"=w176:string)  [unwired: 3 in]
                n233 = Concatenate Strings("D:\\data\\", w176) -> (w177:string)
                n234 = Less?(x="OD num", y=100.0) -> (x < y?=w190:bool)
                n235 = Concatenate Strings(w177, w184) -> (w178:string)
                n236 = case shown="True" w190 {
                  tunnel: "OD num" -> [w201 w203]
                  tunnel: [w200 w202] -> w191
                  frame False {
                    n237 = Number To Decimal String(number=w201) -> (decimal integer string=w200:string)  [unwired: 1 in]
                  }
                  frame True {
                    n238 = Less?(x=w203, y=10.0) -> (x < y?=w204:bool)
                    n239 = case shown="False" w204 {
                      tunnel: w203 -> [w208 w213]
                      tunnel: [w206 w210] -> w202
                      frame False {
                        n240 = Number To Decimal String(number=w208) -> (decimal integer string=w207:string)  [unwired: 1 in]
                        n241 = Concatenate Strings("0" ("字符串"), w207) -> (w206:string)
                      }
                      frame True {
                        n242 = Number To Decimal String(number=w213) -> (decimal integer string=w211:string)  [unwired: 1 in]
                        n243 = Concatenate Strings("00" ("字符串"), w211) -> (w210:string)
                      }
                    }
                  }
                }
                n244 = Concatenate Strings(w178, w179) -> (w180:string)
                n245 = Concatenate Strings(w180, w184) -> (w181:string)
                n246 = Concatenate Strings(w181, w182) -> (w183:string)
                n247 = Concatenate Strings(w183, w184) -> (w185:string)
                n248 = Concatenate Strings(w185, w191) -> (w186:string)
                n249 = Concatenate Strings(w186, "-OD" ("字符串")) -> (w188:string)
                n250 = String To Path(string=w188) -> (path=w197:path)
                n251 = local write "From OD fit?"(TRUE ("From OD fit?")) -> ()
                n252 = local write "OD fit"(FALSE ("OD fit")) -> ()
                n253 = call "IMAQ Create"("Image Name"="untitled", "Image Type"=w193) -> ("New Image"=w198:T3)  [unwired: 3 in, 1 out]
                n254 = call <vilib>:"Open a Document on Disk.vi"("document path"=w197) -> ()  [unwired: 6 in, 1 out]
                n255 = call "IMAQ ReadFile"("File Path"=w197, "Image"=w198) -> ("Image Out"=w199:T3)  [unwired: 5 in, 4 out]
                n256 = call "IMAQ ImageToArray"("Image"=w199) -> ("Image Pixels (U16)"=w195:u16[][], "error out"=w194:errorcluster)  [unwired: 3 in, 3 out]
                n257 = local write "Latest image data"(w195) -> ()
                n258 = local write "OD image"(w195) -> ()
                n259 = call "IMAQ Dispose"("Image"=w199, "error in (no error)"=w194) -> ()  [unwired: 4 in, 1 out]
              }
              frame "INI" {
                w218 = 1 items=["FreeRunning", "LockNext", "LockLatest"] ("mode")
                # "Setup Camera Index"
                # "Set grab mode"
                # "Make Sure the camera is not running"
                n260 = property class="IActiveFlyCapControl"(reference=w214, "Camera"=0 ("Start")) -> (reference out=w219:refnum<k7>)  [unwired: 1 in, 1 out]
                n261 = invoke class="IActiveFlyCapControl" method="ShowCamSlnModal"(reference=w219) -> (reference out=w222:refnum<k7>)  [unwired: 2 in, 2 out]
                n262 = property class="IActiveFlyCapControl"(reference=w222, "Start"=0 ("Camera")) -> (reference out=w223:refnum<k7>)  [unwired: 1 in, 1 out]
                n263 = invoke class="IActiveFlyCapControl" method="SetGrabMode"(reference=w223, "mode"=w218) -> (reference out=w215:refnum<k7>)  [unwired: 2 in, 3 out]
                n264 = local write "Initialize"(FALSE ("Initialize")) -> ()
                n265 = property on="Camera Config" class="Bool (strict)"("DisabledEnum"=T1."Enabled" ("禁用")) -> ()  [unwired: 2 in, 2 out]
                n266 = property on="Aquire" class="Bool (strict)"("DisabledEnum"=T1."Enabled" ("禁用")) -> ()  [unwired: 2 in, 2 out]
              }
              frame "CLE" {
                n267 = for {
                  N: 5 -> [_]
                  tunnel: w228 -> [w230]
                  tunnel: [w229] -> w226
                  n268 = invoke class="IActiveFlyCapControl" method="GrabImage"(reference=w230) -> (reference out=w229:refnum<k7>)  [unwired: 2 in, 2 out]
                }
                n269 = local write "Reset process index"(FALSE ("Reset process index")) -> ()
              }
            }
          }
        }
      }
    }
    frame #2 {
      n270 = Release Queue(queue=w403) -> ()  [unwired: 2 in, 3 out]
      n271 = Release Queue(queue=w405) -> ()  [unwired: 2 in, 3 out]
      n272 = Release Queue(queue=w404) -> ()  [unwired: 2 in, 3 out]
    }
  }
